vi "RSNRPZ Set Trigger Level.vi"(8 "error in (no error)":errorcluster, 9 "Trigger Level (1.0e-6 W)":dbl=1e-06 format="%.2p", 10 "Channel (1)":i32=1, 11 "VISA session":refnum<visa-resource-name> caption="VISA resource name") -> (0 "error out":errorcluster, 3 "dup VISA session":refnum<visa-resource-name> caption="VISA resource name")   [LabVIEW 2010]
doc: "This VI determines the power a trigger signal must exceed before a trigger event is detected. This setting is only used for internal trigger signal source.\n\nRemote-control command(s):\nTRIG:LEV"
uses:
  rsnrpz_32.dll
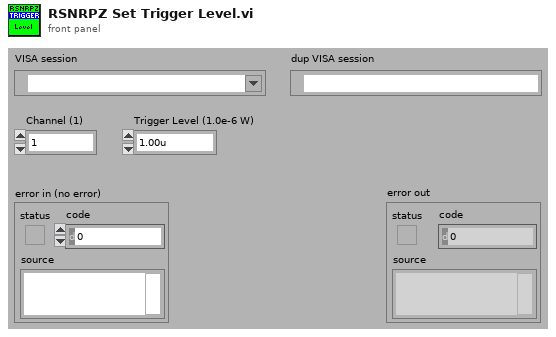
[diagram p1: front panel]
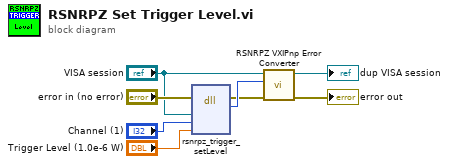
[diagram p0: block diagram]
diagram:
  n1 = dll-call lib="rsnrpz_32.dll" fn="rsnrpz_trigger_setLevel"(error in="error in (no error)", "VISA Session"="VISA session", "Channel"="Channel (1)", "Trigger Level"="Trigger Level (1.0e-6 W)") -> (error out=w5:errorcluster, "Status"=w8:i32)  [unwired: 5 in, 1 out]
  n2 = call <instrlib>:"RSNRPZ VXIPnp Error Converter.vi"("error in"=w5, "VXIPnp error code"=w8, "VISA session"="VISA session") -> ("error out"=→"error out":errorcluster, "dup VISA session"=→"dup VISA session":refnum<visa-resource-name>)  [unwired: 7 in]
